vi "Screen Capture.vi"(8 "error in (no error)":errorcluster, 9 "Dest Filename":path, 11 "VISA resource name":refnum<visa-resource-name>) -> (0 "error out":errorcluster, 3 "VISA resource name out":refnum<visa-resource-name>)   [LabVIEW 2013, in "LeCroy Wave Series.lvlib"]
doc: "Transfers a file from the oscilloscope's hard drive to a destination filepath on the remote PC. If the destination filename already exists, then the file isn't saved."
uses:
  LeCroy Wave Series.lvlib
panel:
  in  "Color (0: Standard)":enum16{"Standard", "Print", "Black & White"}(ring)
  in  "Hardcopy area (1: DSOWINDOW)":T1(ring)
  in  "Filetype (0: BMP)":T2(ring)
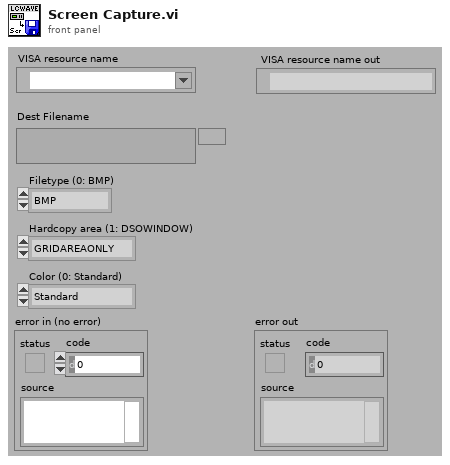
[diagram p1: front panel]
types:
  T1 = enum16{"GRIDAREAONLY", "DSOWINDOW", "FULLSCREEN"}
  T2 = enum16{"BMP", "BMPCOMP", "JPEG", "PNG", "TIFF", "PSD"}
  T3 = enum16{"open", "open or create", "create or replace", "create", "open (read only)"}
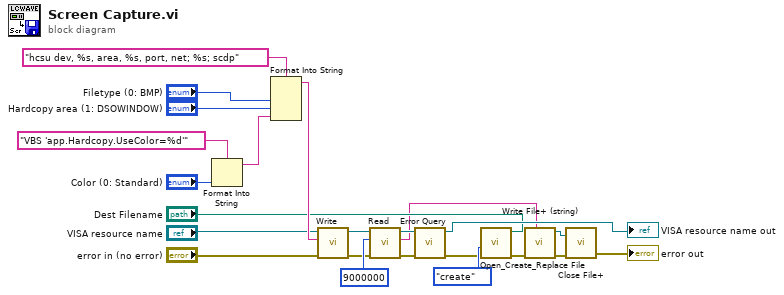
[diagram p0: block diagram]
diagram:
  n1 = Format Into String(format string="VBS 'app.Hardcopy.UseColor=%d'", "Color (0: Standard)") -> (resulting string=w10:string)  [unwired: 2 in, 1 out]
  n2 = Format Into String(format string="hcsu dev, %s, area, %s, port, net; %s; scdp" ("Write Buffer"), "Filetype (0: BMP)", "Hardcopy area (1: DSOWINDOW)", w10) -> (resulting string=w15:string)  [unwired: 2 in, 1 out]
  n3 = call "Write.vi"("error in (no error)"="error in (no error)", "Write Buffer"=w15, "VISA resource name"="VISA resource name") -> ("error out"=w21:errorcluster, "VISA resource name out"=w22:refnum<visa-resource-name>)  [unwired: 6 in, 1 out]
  n4 = call "Read.vi"("error in (no error)"=w21, "Byte Count"=u32 9000000, "VISA resource name"=w22) -> ("error out"=w19:errorcluster, "Read Buffer"=w5:string, "VISA resource name out"=w18:refnum<visa-resource-name>)  [unwired: 5 in, 1 out]
  n5 = call "Error Query.vi"("error in (no error)"=w19, "VISA resource name"=w18) -> ("error out"=w4:errorcluster, "VISA resource name out"=→"VISA resource name out":refnum<visa-resource-name>)  [unwired: 6 in, 2 out]
  n6 = call <vilib>:"Open_Create_Replace File.vi"("error in (no error)"=w4, "function (open:0)"=T3."create", "file path"="Dest Filename") -> ("error out"=w7:errorcluster, "refnum"=w2:refnum<file>)  [unwired: 5 in, 2 out]
  n7 = call <vilib>:"Write File+ (string).vi"("string"=w5, "error in (no error)"=w7, "refnum"=w2) -> ("error out"=w6:errorcluster, "dup refnum"=w1:refnum<file>)  [unwired: 4 in, 1 out]
  n8 = call <vilib>:"Close File+.vi"("error in (no error)"=w6, "refnum"=w1) -> ("error out"=→"error out":errorcluster)  [unwired: 3 in, 2 out]
